vi "LLMain.vi"() -> ()   [LabVIEW 2009]
uses:
  LinkedList.lvclass
  LLSearch/LLSearch.lvclass
  LLNode/LLNode.lvclass
  InsertSearch.ctl
  position.ctl
  RemoveSearch.ctl
panel:
  out "LinkedList out":refnum<class "LinkedList.lvclass">
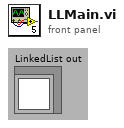
[diagram p1: front panel]
types:
  T1 = typedef "LinkedList.lvclass/position.ctl" = enum16{"Front", "Back", "Search"}
  T2 = typedef "LinkedList.lvclass/InsertSearch.ctl" = cluster{"LLSearch in":refnum<class "LLSearch.lvclass">, "InsertIfEmpty":bool, "Insert After":bool, "InsertIfNotFound":bool}
  T3 = typedef "LinkedList.lvclass/RemoveSearch.ctl" = cluster{"LLSearch":refnum<class "LLSearch.lvclass">, "length":u32}
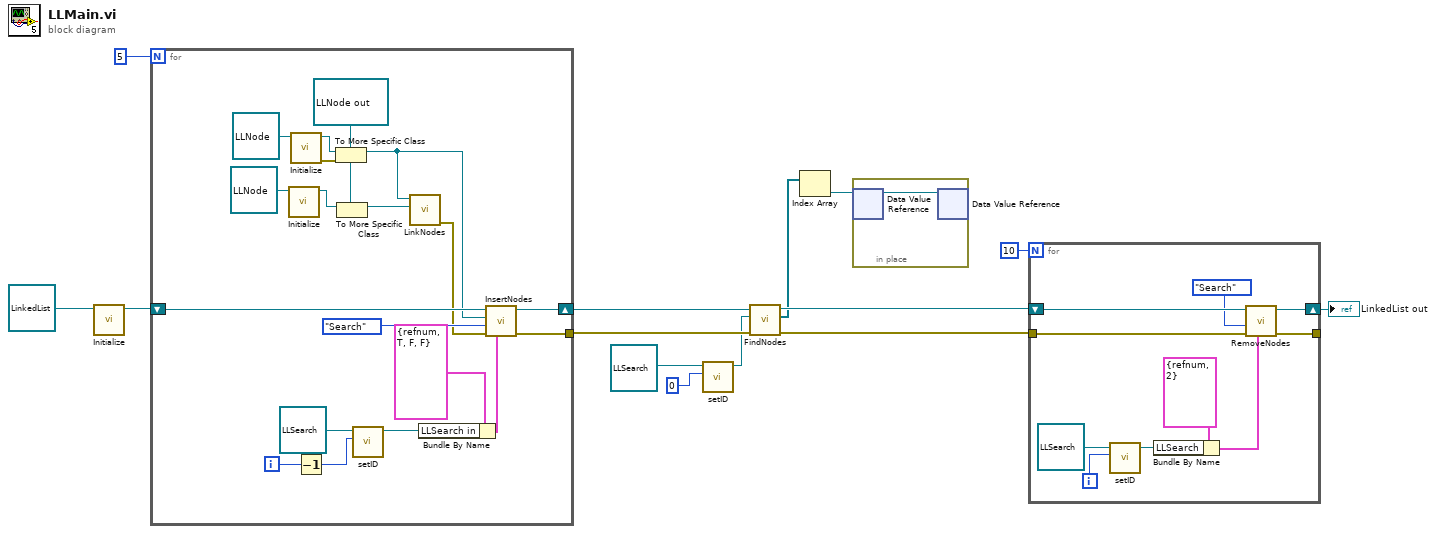
[diagram p0: block diagram]
diagram:
  n1 = call-dynamic "Initialize.vi"("LinkedList in"=refnum<class "LinkedList.lvclass"> refnum ("LinkedList.lvclass")) -> ("LinkedList out"=w13:refnum<class "LinkedList.lvclass">)  [unwired: 9 in, 1 out]
  n2 = for {
    N: 5 -> [_]
    shift-right: [w30] -> w7
    shift-left: w13 -> [w29]
    tunnel: [w27] -> w4
    i -> [w18]
    w28 = refnum<data-value> refnum ("ToInsert")
    n3 = call-dynamic "Initialize.vi"("LLNode data"=refnum<class "LLNode.lvclass"> refnum ("LLNode.lvclass")) -> ("Node out"=w16:refnum<data-value>)  [unwired: 9 in, 1 out]
    n4 = call-dynamic "Initialize.vi"("LLNode data"=refnum<class "LLNode.lvclass"> refnum ("LLNode.lvclass")) -> ("error out"=w32:errorcluster, "Node out"=w31:refnum<data-value>)  [unwired: 9 in]
    n5 = Decrement(x=w18) -> (x-1=w19:i32)
    n6 = To More Specific Class(target class=w28, reference=w31, error in=w32) -> (specific class reference=w26:refnum<data-value>)  [unwired: 1 out]
    n7 = To More Specific Class(target class=w28, reference=w16) -> (specific class reference=w15:refnum<data-value>)  [unwired: 1 in, 1 out]
    n8 = call "setID.vi"("ID"=w19, "LLSearch in"=refnum<class "LLSearch.lvclass"> refnum) -> ("LLSearch out"=w23:refnum<class "LLSearch.lvclass">)  [unwired: 8 in, 1 out]
    n9 = call "LinkNodes.vi"("NextNode in"=w15, "PreviousNode in"=w26) -> ("error out"=w21:errorcluster)  [unwired: 7 in, 2 out]
    n10 = Bundle By Name(cluster=T2 {"LLSearch in"=refnum, "InsertIfEmpty"=TRUE, "Insert After"=FALSE, "InsertIfNotFound"=FALSE} ("Insert Search"), "LLSearch in"=w23) -> (w22:T2)
    n11 = call "InsertNodes.vi"("Insert Search"=w22, "error in (no error)"=w21, "position"=position."Search", "ToInsert"=w26, "LinkedList in"=w29) -> ("error out"=w27:errorcluster, "LinkedList out"=w30:refnum<class "LinkedList.lvclass">)  [unwired: 4 in, 1 out]
  }
  n12 = call "setID.vi"("ID"=u32 0, "LLSearch in"=refnum<class "LLSearch.lvclass"> refnum ("LLSearch")) -> ("LLSearch out"=w3:refnum<class "LLSearch.lvclass">)  [unwired: 8 in, 1 out]
  n13 = call "FindNodes.vi"("error in (no error)"=w4, "Search"=w3, "LinkedList in"=w7) -> ("error out"=w5:errorcluster, "LLNodes"=w2:refnum<data-value>[], "LinkedList out"=w6:refnum<class "LinkedList.lvclass">)  [unwired: 5 in, 1 out]
  n14 = Index Array(array=w2) -> (element=w1:refnum<data-value>)  [unwired: 1 in]
  n15 = in-place {
    n16 = in-place-dvr #1(w1) -> (w34:refnum<class "LLNode.lvclass">)  [unwired: 1 out]
    n17 = in-place-dvr #1(w34) -> ()  [unwired: 2 out]
  }
  n18 = for {
    N: 10 -> [_]
    shift-right: [w43] -> w10
    shift-left: w6 -> [w44]
    tunnel: w5 -> [w42]
    tunnel: [w40] -> _
    i -> [w38]
    n19 = call "setID.vi"("ID"=w38, "LLSearch in"=refnum<class "LLSearch.lvclass"> refnum ("LLSearch")) -> ("LLSearch out"=w36:refnum<class "LLSearch.lvclass">)  [unwired: 8 in, 1 out]
    n20 = Bundle By Name(cluster=T3 {"LLSearch"=refnum, "length"=2} ("RemoveSearch"), "LLSearch"=w36) -> (w35:T3)
    n21 = call "RemoveNodes.vi"("RemoveSearch"=w35, "error in (no error)"=w42, "position"=position."Search", "LinkedList in"=w44) -> ("error out"=w40:errorcluster, "LinkedList out"=w43:refnum<class "LinkedList.lvclass">)  [unwired: 4 in, 2 out]
  }
  "LinkedList out" <- w10
